vi "Color Picker_File Read Write Color Array.vi"(6 "Read(f)\nWrite(t)":bool, 8 "Error":errorcluster, 9 "Home Path":path, 11 "Template Select":u32[](array[colorbox])) -> (0 "Error Out":errorcluster, 2 "Final Path Out":path, 3 "Template Select Out":u32[](array[colorbox]))   [LabVIEW 2009]
doc: "Reads or Writes the Color history file"
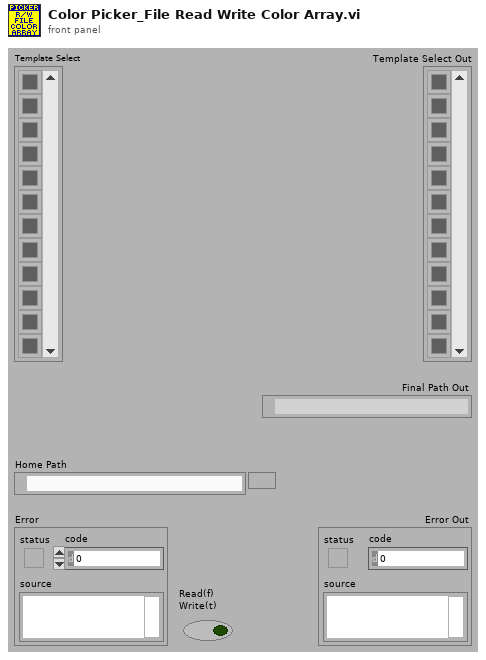
[diagram p1: front panel]
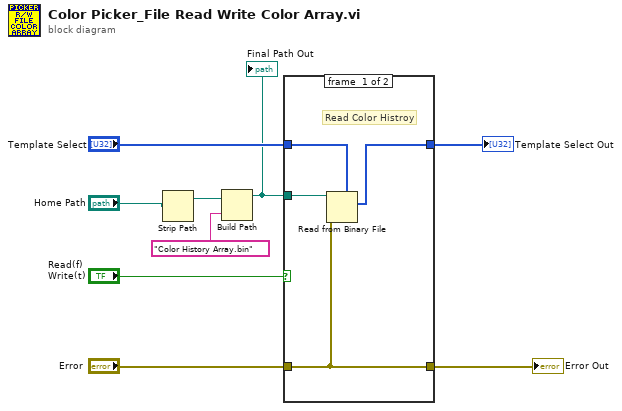
[diagram p0: block diagram]
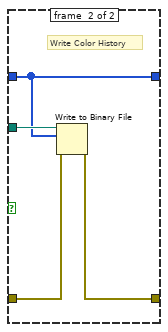
[diagram p2: hidden frame]
diagram:
  n1 = Strip Path(path="Home Path") -> (stripped path=w3:path)  [unwired: 1 out]
  n2 = Build Path(base path=w3, name or relative path="Color History Array.bin") -> (appended path=w5:path)
  "Final Path Out" <- w5
  n3 = case shown="True" "Read(f)\nWrite(t)" {
    tunnel: [w10 w17] -> w9
    tunnel: "Error" -> [w10 w16]
    tunnel: "Template Select" -> [w12 w14]
    tunnel: w5 -> [w13 w15]
    tunnel: [w11 w14] -> w1
    frame #0 {
      # "Read Color Histroy"
      n4 = Read from Binary File(5:w12, 8:w10, 11:w13) -> (2:w11:u32[])  [unwired: 3 in, 3 out]
    }
    frame #1 {
      # "Write Color History"
      n5 = Write to Binary File(file (use dialog)=w15, data=w14, error in=w16) -> (error out=w17:errorcluster)  [unwired: 3 in, 2 out]
    }
  }
  "Error Out" <- w9
  "Template Select Out" <- w1
